vi "Set Scan Engine Sync to Scan.vi"(8 "error in":errorcluster, 10 "sync to scan":bool, 11 "scan engine custom device ref in":T1 format="%.0x") -> (0 "error out":errorcluster, 3 "scan engine custom device ref out":T1 format="%.0x")   [LabVIEW 2017, in "Scan Engine Scripting.lvlib"]
uses:
  Scan Engine Scripting.lvlib
  <vilib>/NI Veristand/Custom Device API/Custom Device Item Ref.ctl
  Scan Engine Custom Device.lvlib
  <vilib>/NI Veristand/Custom Device API/Custom Device API.lvlib
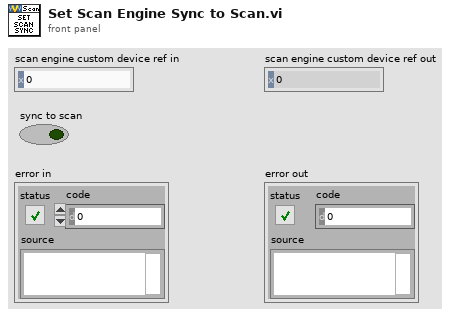
[diagram p1: front panel]
types:
  T1 = typedef "Custom Device API.lvlib/Custom Device Item Ref.ctl" = u64
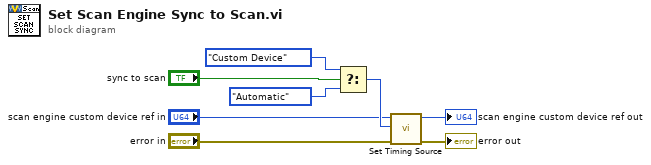
[diagram p0: block diagram]
diagram:
  n1 = Select(t=enum16{"Automatic", "Custom Device"}."Custom Device" ("Timing Source"), s="sync to scan", f=enum16{"Automatic", "Custom Device"}."Automatic" ("Timing Source")) -> (s? t:f=w5:enum16{"Automatic", "Custom Device"})
  n2 = call "Set Timing Source.vi"("error in (no error)"="error in", "Timing Source"=w5, "Item Ref in"="scan engine custom device ref in") -> ("error out"=→"error out":errorcluster, "Item Ref out"=→"scan engine custom device ref out":T1)  [unwired: 7 in]
